vi "play-general-scan.vi"() -> ()   [LabVIEW 2017]
uses:
  fpga_VIs/fpga_subVIs_ssxy/fixed-point-ss/typeDefs/FXPControlParams-ss-xy.ctl
  controls/z-axis-params_v4_prescan.ctl
  controls/TF-params.ctl
  controls/scan_input_meta_data.ctl
  controls/scan-mode-CTL.ctl
  fpga_VIs/controls/supervisor-params.ctl
  fpga_VIs/controls/fpga-scan-status.ctl
  controls/boolean_info.ctl
  controls/auto_id_result.ctl
  subVIs/auto-sys-id/controls/SOS_frf_data.ctl
  fpga_interface_lib/fpga_interface_types/cs-scan-inputs-TYPE.ctl
  <vilib>/userdefined/High Color/nirio_resource_hc.ctl
  controls/rasterMetaData_asCS.ctl
  <vilib>/FPGAPlugInAG/cRIO-9082/niLvFpga_Open_cRIO-9082.vi
  <vilib>/rvi/interface/common/dynamic/niFpgaDynamicAddResources.vi
  <vilib>/FPGAPlugInAG/Dynamic/niLvFpga_Reset_Dynamic.vi
  <vilib>/Utility/error.llb/Error Cluster From Error Code.vi
  <vilib>/rvi/errors/niLvFpgaAdjustHostInterfaceError.vi
  <vilib>/FPGAPlugInAG/Dynamic/niLvFpga_Run_Dynamic.vi
  fpga_interface_lib/acquire_FXP_16-5_FIFO_2.vi
  <vilib>/RVI Host/nirviSupport.llb/nirviErrorClusterFromErrorCode.vi
  <vilib>/FPGAPlugInAG/Dynamic/niLvFpga_Close_Dynamic.vi
  <vilib>/rvi/interface/nirviOpenFPGA/nirviOpenFPGA.xnode
  FPGA Bitfiles/afmimagingcontro_FPGATargetSPARTA_cs-scanningv5ssx.lvbitx
  <vilib>/rvi/interface/nirviMethod/nirviMethod.xnode
  <vilib>/rvi/interface/nirviReadWriteControl/nirviReadWriteControl.xnode
  <vilib>/rvi/interface/nirviCloseFPGA/nirviCloseFPGA.xnode
  <vilib>/rvi/interface/Simulation/niFpgaSimulationCallBeginRW.vi
  NiFpgaLv.dll
  fpga_interface_lib/fpga_interface.lvlib
  <vilib>/addons/_JKI.lib/Serialization/JSON/JKI JSON Serialization.lvlib
  <vilib>/rvi/interface/nirviMethod/StockFPGA_InlinedMethodWaitForSingleIRQ.vi
  <vilib>/FPGAPlugInAG/Dynamic/niLvFpga_WaitOnIrq_Dynamic.vi
  <vilib>/FPGAPlugInAG/Dynamic/niLvFpga_AcknowledgeIrq_Dynamic.vi
  labview/utils_lib/utils.lvlib
panel:
  in  "enable-gdriftX":bool
  in  "enable-Dx":bool
  out "current-state":u8
  out "uy_k":fxp<+/-,32,5>
  in  "Ki-y":sgl=0.01
  in  "enable-Dy":bool=TRUE
  in  "Array 5":path[](array[path])
  out "size(s)":i32
  in  "log-channels":u16(ring)=6 items=["without-friction"=5, "with-friction"=6]
  in  "lpf-enable":bool=TRUE
  out "Array 3":T1(array[cluster])
  out "current-scan number":i32
  out "state0-count":u64
  out "output cluster":T2={"xy_settled_samples_threshold"=15, "xy_error_threshold"=0.01, "zup_err_threshold"=0.10000228881835938, "prescan_samples"=5000, "TOL"=0.3, "collect_all"=TRUE, "numEntities"=0} {"TOL" format="%#_13g"}
  out "error out":errorcluster
  in  "Alert-on-Finish":bool
  out "state times":dbl[](array[numeric])
  in  "Tab Control":T3(tab)
  in  "z_axis_params":T4={"z_u_max"=2.0, "setpoint_scan"=-0.3000030517578125, "Ki_scan"=0.07, "uz_safe"=0.2998046875, "Kiz_down"=0.045, "setpoint_up"=-0.8000030517578125, "do_Dz"=TRUE, "PID_while_xy_move"=FALSE, "TF_params"={"TF_order"=2, "Num"=[1.0, -1.9962076, 0.9990926, 0.0, 0.0, 0.0, 0.0, 0.0, 0.0], "Den"=[1.0, -1.9961313, 0.9990842, 0.0, 0.0, 0.0, 0.0, 0.0, 0.0]}, "KI_slope"=1.0, "enable_KI_sched"=FALSE, "KI_min"=0.0099945068359375, "KI_max"=0.1999969482421875} {"Kiz_down" format="%#_13g"; "Ki_scan" min=0 max=0.4 step=0.0025; "z_u_max" format="%#_13g"}
  in  "overwrite":bool
  in  "note-blob":string
  in  "state-machine-params":T2={"xy_settled_samples_threshold"=20, "xy_error_threshold"=0.01, "zup_err_threshold"=0.05100059509277344, "prescan_samples"=0, "TOL"=0.0259, "collect_all"=TRUE, "numEntities"=0} {"TOL" format="%#_13g"}
  in  "trigger-0":bool
  in  "STOP":bool
  out "CS Time":dbl
  in  "collect-0":bool
  in  "Continue":bool
  out "output-data-paths":path[](array[path])
  in  "file path (use dialog)":path=path "C:/Users/arnold/Documents/afm-cs/labview/first_res_fit_current.json"
  in  "xy-gain-mult":dbl=1.0 min=0.0 max=1.0 step=1.0 format="%#_13g"
  out "current-input-file":string
  in  "control_data_path":path=path "Z:/afm-cs/step-exps/LinControls-choose-zeta_5micron_xyff.json"
  in  "umax-xy":dbl=5.0 format="%#_13g"
  out "ControlParamsLin-ss":T6={"umax"=3.0, "Ns_obs/cntrl"=0, "du_max"=0.0, "Nbar"=0.0, "Nhyst"=0, "Nsat"=0, "Ndrift+1"=0, "Ki-y"=0.01, "Ns_xff+1"=0, "Ns_yff+1"=0, "Ns_Dx+1"=0, "Ns_Dy+1"=0, "Ki-x"=0.01}
  out "scan-status":T7
  out "error out 2":errorcluster
  out "scan_meta":T9
  out "Kiscan-effective":dbl
  out "Kidown-effective":dbl
  out "K":dbl
  out "last-state":u8[](array[numeric])
  out "Z-RESONANCE":T11
  out "input-file-check":bool[](array[boolean])
  out "output-meta-data-path":path
  # "C:\\Users\\arnold\\Documents\\afm-cs\\labview\\first_res_fit-4-19-2019-sicon.json"
  # "make this come from input csv!"
  # "For the y-axis only, shouldnt ever really\nneed to change"
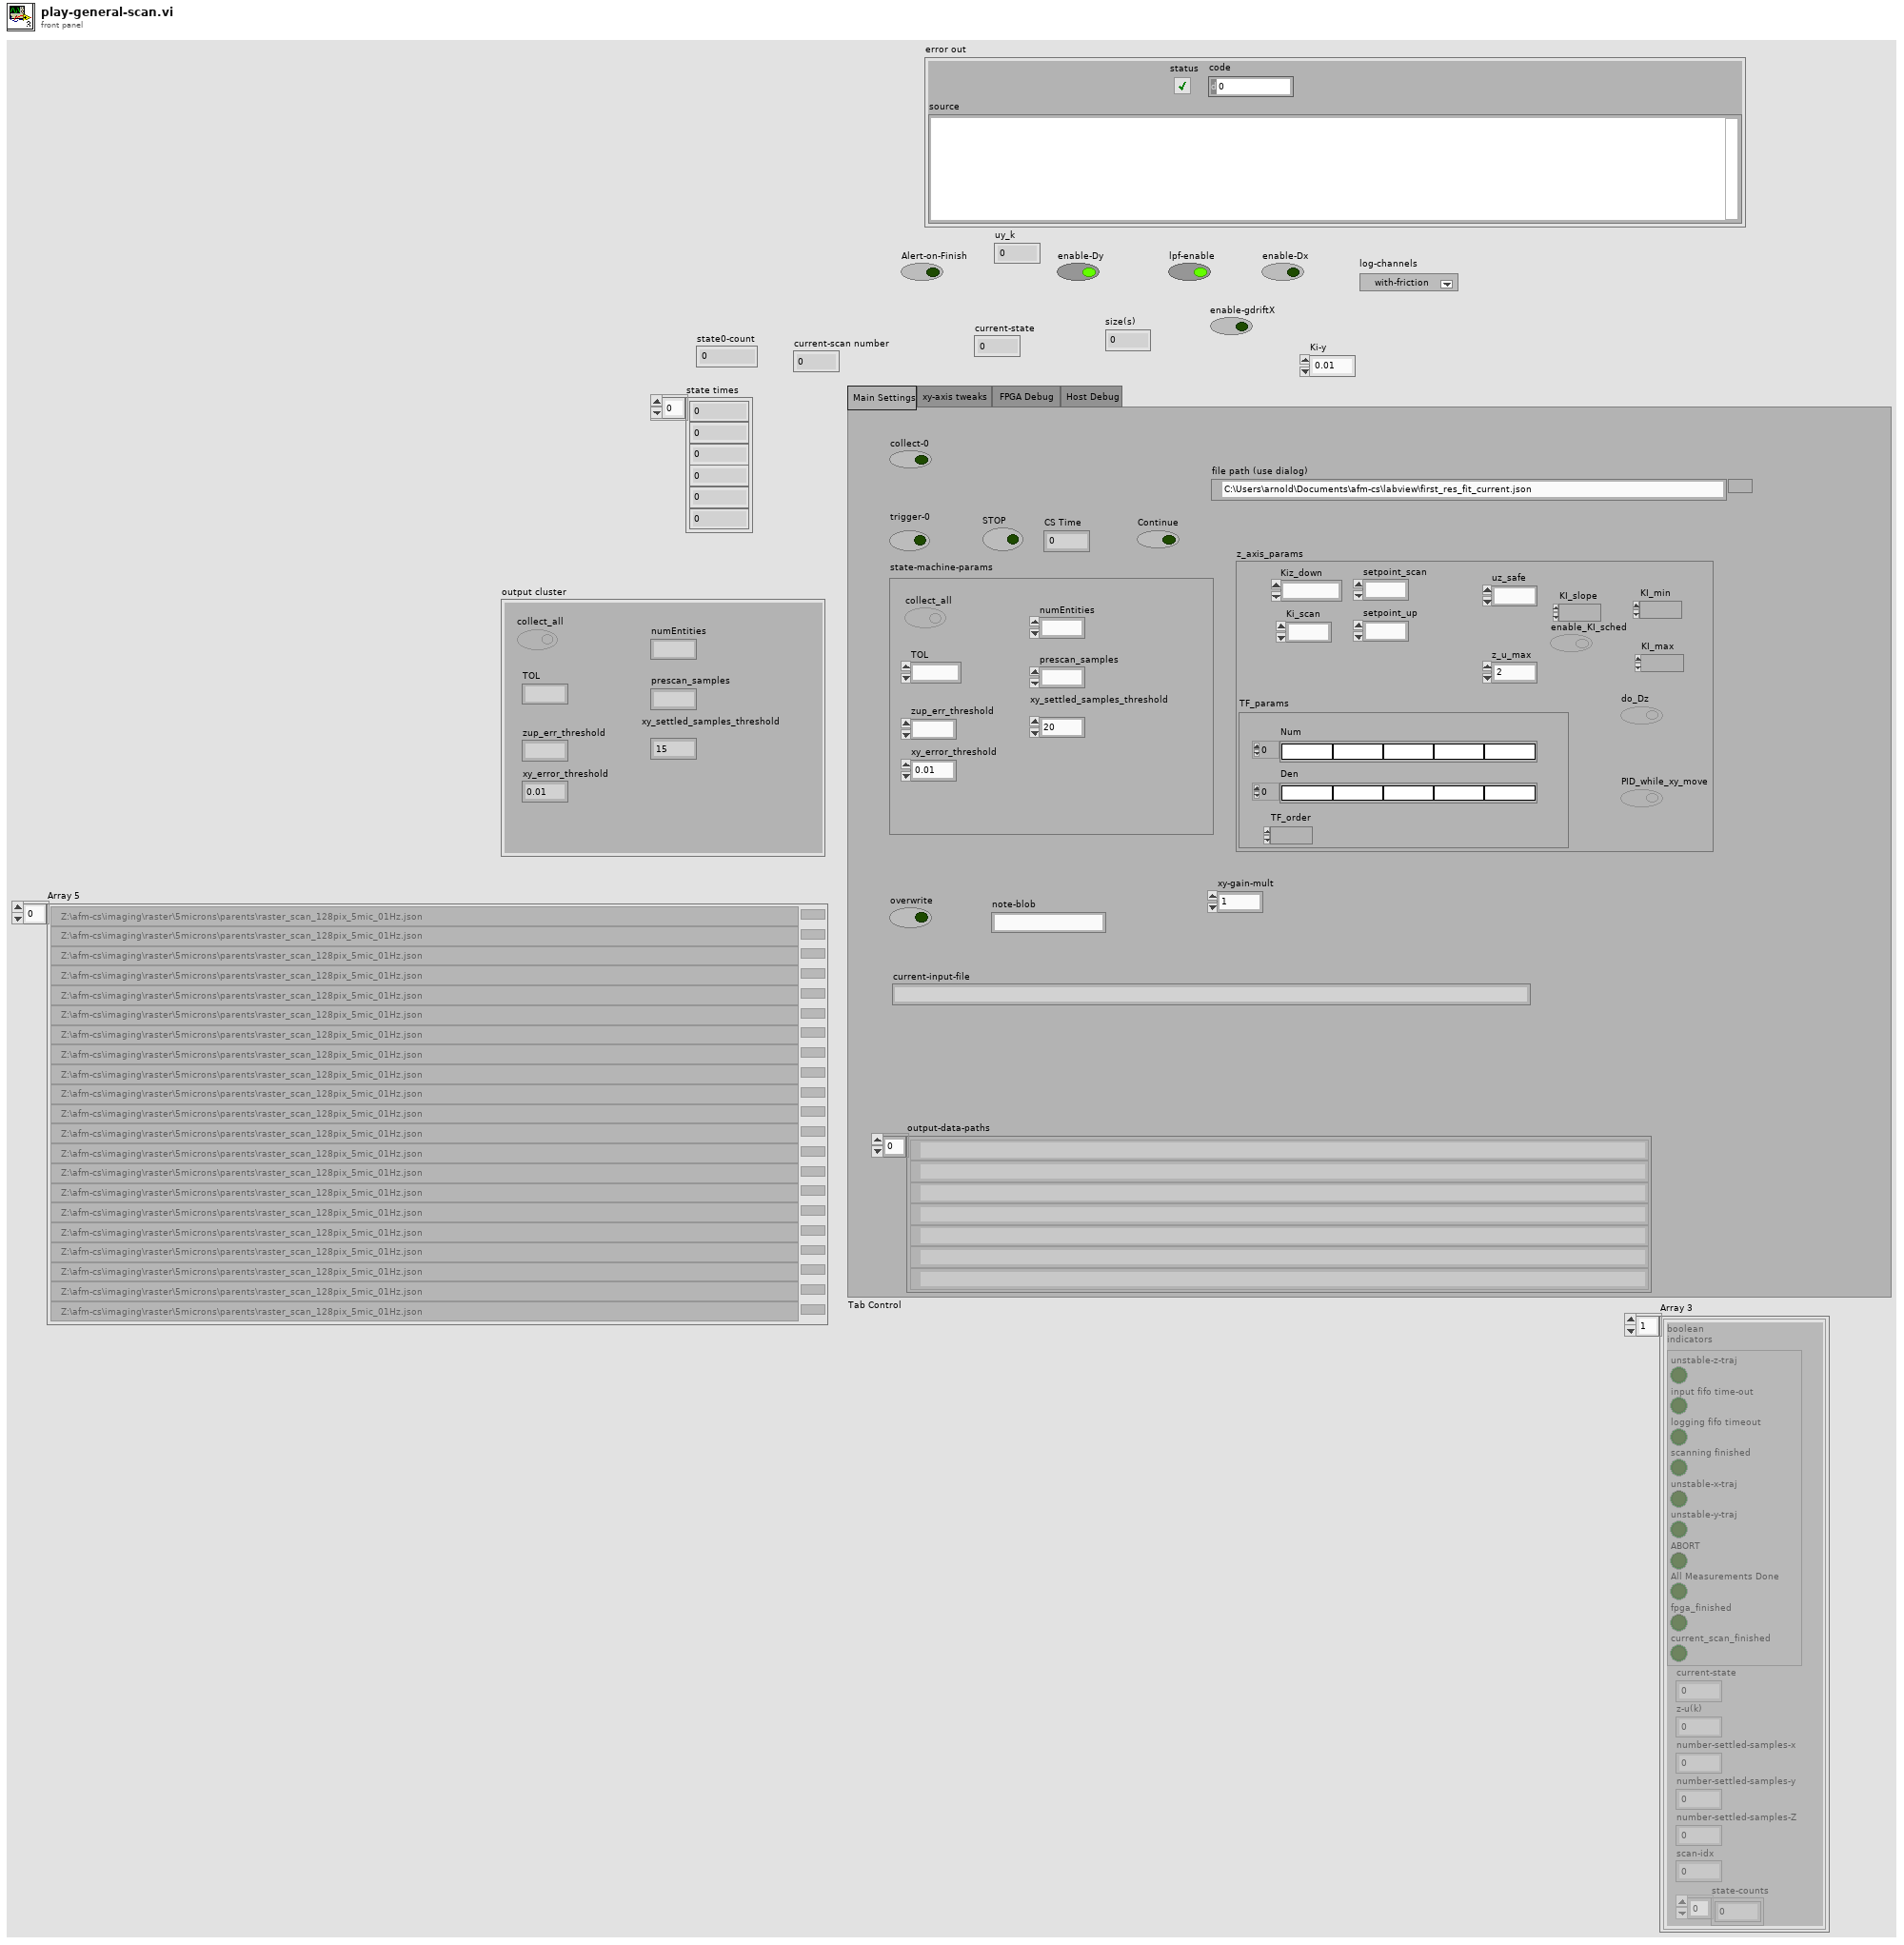
[diagram p1: front panel]
types:
  T1 = cluster{"boolean \nindicators":cluster{"unstable-z-traj":bool, "input fifo time-out":bool, "logging fifo timeout":bool, "scanning finished":bool, "unstable-x-traj":bool, "unstable-y-traj":bool, "ABORT":bool, "All Measurements Done":bool, "fpga_finished":bool, "current_scan_finished":bool}, "current-state":u8, "z-u(k)":sgl, "number-settled-samples-x":i16, "number-settled-samples-y":i16, "number-settled-samples-Z":i16, "scan-idx":i16, "state-counts":u64[]}[]
  T2 = typedef "supervisor-params.ctl" = cluster{"xy_settled_samples_threshold":i16, "xy_error_threshold":sgl, "zup_err_threshold":fxp<+,24,5>, "prescan_samples":i16, "TOL":sgl, "collect_all":bool, "numEntities":i16}
  T3 = enum32{"Main Settings", "xy-axis tweaks", "FPGA Debug ", "Host Debug"}
  T4 = typedef "z-axis-params_v4_prescan.ctl" = cluster{"z_u_max":sgl, "setpoint_scan":fxp<+/-,32,16>, "Ki_scan":sgl, "uz_safe":fxp<+/-,16,5>, "Kiz_down":sgl, "setpoint_up":fxp<+/-,32,16>, "do_Dz":bool, "PID_while_xy_move":bool, "TF_params":T5, "KI_slope":fxp<+/-,32,16>, "enable_KI_sched":bool, "KI_min":fxp<+/-,32,16>, "KI_max":fxp<+/-,32,16>}
  T5 = typedef "TF-params.ctl" = cluster{"TF_order":i16, "Num":sgl[], "Den":sgl[]}
  T6 = typedef "FXPControlParams-ss-xy.ctl" = cluster{"umax":fxp<+/-,18,5>, "Ns_obs/cntrl":u8, "du_max":fxp<+/-,18,5>, "Nbar":fxp<+/-,32,5>, "Nhyst":u8, "Nsat":u8, "Ndrift+1":u8, "Ki-y":sgl, "Ns_xff+1":u8, "Ns_yff+1":u8, "Ns_Dx+1":u8, "Ns_Dy+1":u8, "Ki-x":sgl}
  T7 = typedef "fpga-scan-status.ctl" = cluster{"boolean \nindicators":T8, "current-state":u8, "z-u(k)":sgl, "number-settled-samples-x":i16, "number-settled-samples-y":i16, "number-settled-samples-Z":i16, "scan-idx":i16, "state-counts":u64[]}
  T8 = typedef "boolean_info.ctl" = cluster{"unstable-z-traj":bool, "input fifo time-out":bool, "logging fifo timeout":bool, "scanning finished":bool, "unstable-x-traj":bool, "unstable-y-traj":bool, "ABORT":bool, "All Measurements Done":bool, "fpga_finished":bool, "current_scan_finished":bool}
  T9 = typedef "scan_input_meta_data.ctl" = cluster{"npix":i64, "raster_freq":dbl, "width":dbl, "points_per_line":i64, "points_per_period":i64, "total_num_points":i64, "scan_type":T10, "number_of_scans":i64, "actual_sub_samble_perc":dbl, "mu_length":dbl, "tip_velocity":dbl, "pix_idx":i32[], "overscan_samples":i16, "pre_scan_samples":i16}
  T10 = typedef "scan-mode-CTL.ctl" = enum16{"raster", "CS"}
  T11 = typedef "auto_id_result.ctl" = cluster{"Dinv_Num":dbl[], "SOS_frf_data":T12, "Dinv_den":dbl[], "K":dbl}
  T12 = typedef "SOS_frf_data.ctl" = cluster{"omegas":dbl[], "resp_real":dbl[], "resp_imag":dbl[], "theta0":dbl[]}
  T13 = enum16{"open", "replace", "create", "open or create", "replace or create", "replace or create with confirmation"}
  T14 = typedef "fpga_interface.lvlib/cs-scan-inputs-TYPE.ctl" = refnum<k20>
  T15 = typedef "nirio_resource_hc.ctl" = tag
  T16 = typedef "rasterMetaData_asCS.ctl" = cluster{"Ki_xy":dbl, "number_of_lines":i32, "Ki_derate":sgl, "ze_sched_thresh":sgl, "scan_meta":T9, "z_axis_params":T4, "state_counts":dbl[], "state_machine_params":T2, "input_data_path":path, "output_data_path":path, "xy_control_path":path}
  T17 = cluster{"boolean \nindicators":cluster{"unstable-z-traj":bool, "input fifo time-out":bool, "logging fifo timeout":bool, "scanning finished":bool, "unstable-x-traj":bool, "unstable-y-traj":bool, "ABORT":bool, "All Measurements Done":bool, "fpga_finished":bool, "current_scan_finished":bool}, "current-state":u8, "z-u(k)":sgl, "number-settled-samples-x":i16, "number-settled-samples-y":i16, "number-settled-samples-Z":i16, "scan-idx":i16, "state-counts":u64[]}
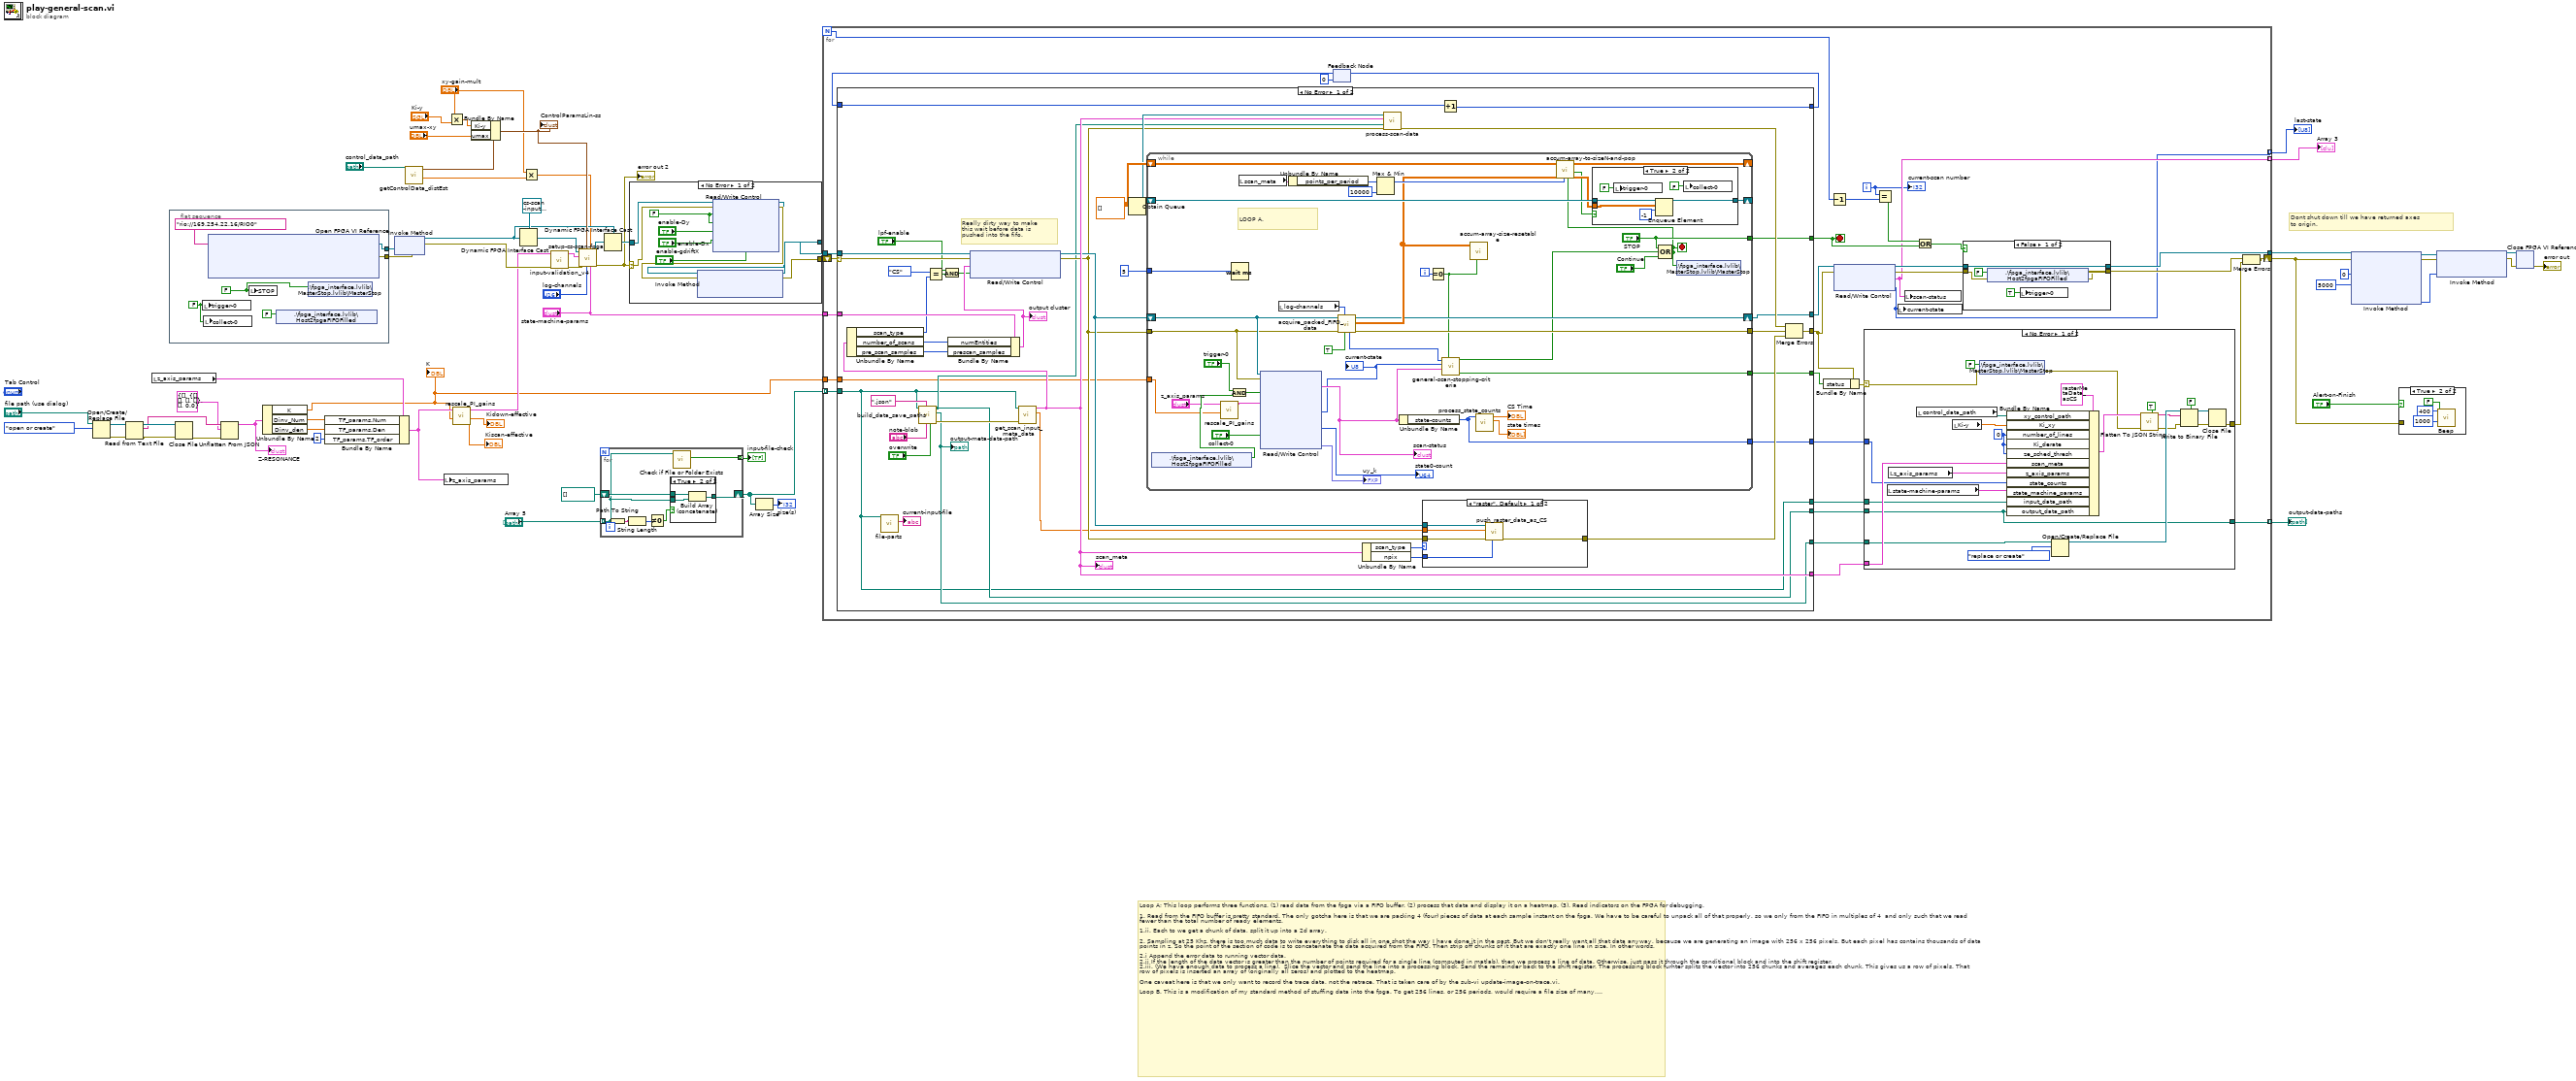
[diagram p0: block diagram]
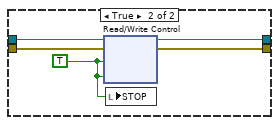
[diagram p4: hidden frame]
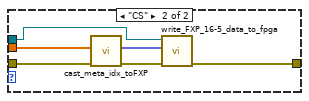
[diagram p6: hidden frame]
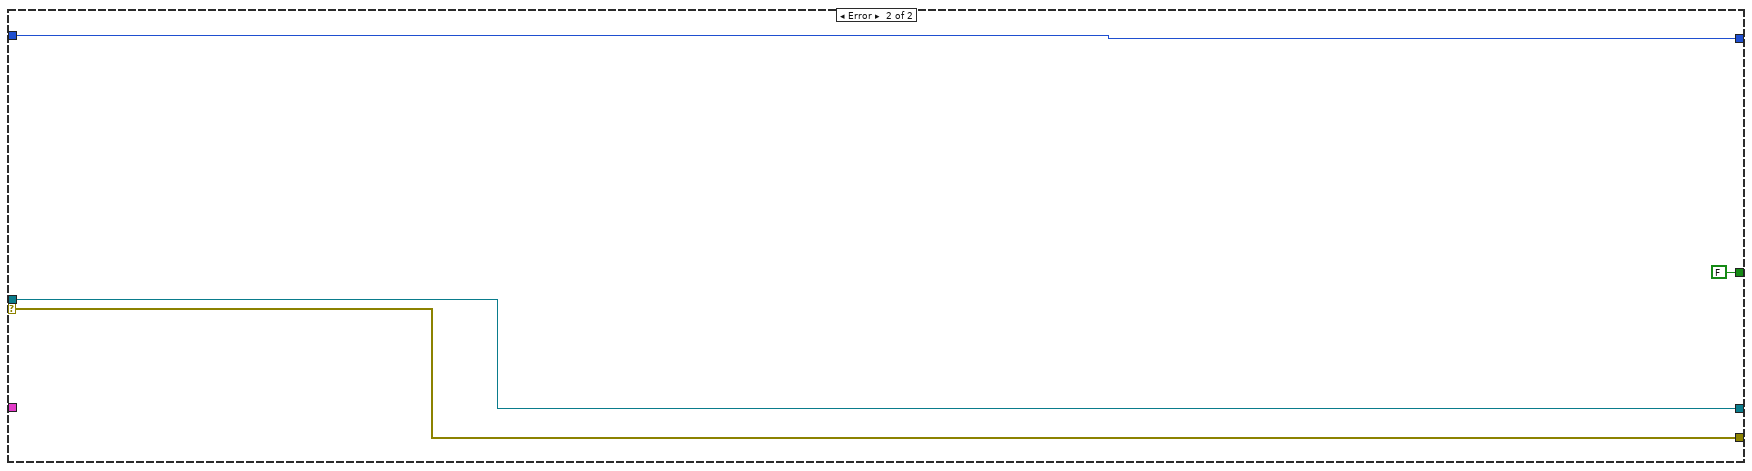
[diagram p8: hidden frame]
diagram:
  # "Dont shut down till we have returned axes\nto origin."
  # "Loop A; This loop performs three functions. (1) read data from the fpga via a FIFO buffer. (2) process that data and display it on a heatmap. (3). Read indicators on the FPGA for debugging.\n\n1. Read from the FIFO buffer is pretty standard. The only gotcha here is that we are packing 4 (four) pieces of data at each sample instant on the fpga. We have to be careful to unpack all of that properly, so we only from the FIFO in multiples of 4  and only such that we read fewer than the total number of ready elements. \n\n1.ii. Each to we get a chunk of data, split it up into a 2d array. \n\n2. Sampling at 25 Khz, there is too much data to write everything to disk all in one shot the way I have done it in the past. But we don't really want all that data anyway, because we are generating an image with 256 x 256 pixels. But each pixel has contains thousands of data points in z. So the point of the section of code is to concatenate the data acquired from the FIFO. Then strip off chunks of it that are exactly one line in size. In other words,\n\n2.i Append the error data to running vector data.\n2.ii If the length of the data vector is greater than the number of points required for a single line (computed in matlab), then we process a line of data. Otherwise, just pass it through the conditional block and into the shift register. \n2.iii. (We have enough data to process a line).  Slice the vector and send the line into a processing block. Send the remainder back to the shift register. The processing block furhter splits the vector into 256 chunks and averages each chunk. This gives us a row of pixels. That row of pixels is inserted an array of (originally all zeros) and plotted to the heatmap.\n\nOne caveat here is that we only want to record the trace data, not the retrace. That is taken care of by the sub-vi update-image-on-trace.vi.\n\nLoop B. This is a modification of my standard method of stuffing data into the fpga. To get 256 lines, or 256 periods, would require a file size of many, many gigibtyes. SO the point here is to only use a single period of the triangle wave and corresponding ramp signal. Everytime we exauhst that data, re-cycle the same data and keep pumping it back in. The one tricky part here is that we have to be careful to shift the original ramp data up by the appropriate amount. We also have to take special care because of how the data is packed from matlab. [x(1), y(1), x(2), y(2)...].\n\nThe first iteration of the loop, we don't push any data in. All we do is get the number of empty elements.\n\nB.1 Each iteration, strip off ' empty elements ' elements from the array and send them to FIFO. \nB.2.i Is the remaining array empty?\nB.2.ii Grab the very last element. We need this"
  n1 = Open/Create/Replace File(file path (use dialog)="file path (use dialog)", operation (0:open)=T13."open or create") -> (refnum out=w34:refnum<file>, error out=w35:errorcluster)  [unwired: 4 in, 1 out]
  n2 = Read from Text File(file (use dialog)=w34, error in=w35) -> (refnum out=w33:refnum<file>, text=w31:string, error out=w32:errorcluster)  [unwired: 2 in, 1 out]
  n3 = local read "z_axis_params"() -> (w23:T4)
  n4 = flat-sequence {
    tunnel: [w68] -> w62
    tunnel: [w67] -> w61
    frame #0 {
      w63 = FALSE ("trigger-0")
      w65 = FALSE
      n5 = local write "trigger-0"(w63) -> ()
      n6 = local write "collect-0"(w63) -> ()
      n7 = xnode "Open FPGA VI Reference"("resource name"=T15 "rio://169.254.22.16/RIO0") -> ("FPGA VI Reference Out"=w68:refnum<k20>, "error out"=w67:errorcluster)  [unwired: 1 in]
      n8 = local write "STOP"(w65) -> ()
      n9 = shared-variable ".\\fpga_interface.lvlib\\Host2fpgaFIFOFilled"(FALSE ("Host2fpgaFIFOFilled")) -> ()  [unwired: 1 in, 1 out]
      n10 = shared-variable ".\\fpga_interface.lvlib\\MasterStop.lvlib\\MasterStop"(w65) -> ()  [unwired: 1 in, 1 out]
    }
  }
  n11 = Close File(refnum=w33, error in=w32) -> (error out=w30:errorcluster)  [unwired: 1 out]
  n12 = Unflatten From JSON(JSON string=w31, type and defaults=T11 {"Dinv_Num"=[], "SOS_frf_data"={"omegas"=[], "resp_real"=[], "resp_imag"=[], "theta0"=[]}, "Dinv_den"=[], "K"=0.0} ("auto_id_result 2"), error in (no error)=w30) -> (value=w27:T11)  [unwired: 4 in, 1 out]
  "Z-RESONANCE" <- w27
  n13 = Unbundle By Name(w27) -> ("K"=w12:dbl, "Dinv_Num"=w22:dbl[], "Dinv_den"=w26:dbl[])
  "K" <- w12
  n14 = Bundle By Name(cluster=w23, "TF_params.Num"=w22, "TF_params.Den"=w26, "TF_params.TF_order"=i16 2) -> (w15:T4)
  n15 = xnode "Invoke Method"("FPGA VI Reference In"=w62, "error in"=w61) -> ("FPGA VI Reference Out"=w21:refnum<k20>, "error out"=w41:errorcluster)
  n16 = call "getControlData_distEst.vi"("system data path"="control_data_path") -> ("AllMatrix"=w11:dbl[], "ControlParams"=w59:T6)  [unwired: 7 in, 2 out]
  n17 = local write "z_axis_params"(w15) -> ()
  n18 = Multiply(x="xy-gain-mult", y="Ki-y") -> (x*y=w9:dbl)
  n19 = call "rescale_PI_gains.vi"("Dinv-k"=w12, "z-axis-params-in"=w15) -> ("Kiscan-effective"=→"Kiscan-effective":dbl, "Kidown-effective"=→"Kidown-effective":dbl, "z-axis-params-out"=w16:T4)  [unwired: 7 in]
  n20 = Bundle By Name(cluster=w59, "Ki-y"=w9, "umax"="umax-xy") -> (w42:T6)
  "ControlParamsLin-ss" <- w42
  n21 = Dynamic FPGA Interface Cast(Session In=T14 refnum ("FPGA Interface in"), Type=w21) -> (Session Out=w44:T14)
  n22 = Multiply(x="xy-gain-mult", y=w11) -> (x*y=w10:dbl[])
  n23 = call "input-validation_v4.vi"("error constant"=w41, "z_axis_params"=w16) -> ("error out"=w25:errorcluster, "z_axis_params-out"=w5:T4)  [unwired: 8 in]
  n24 = call "setup-cs-scan-fpga.vi"("state-machine-params"="state-machine-params", "Control-matrices"=w10, "log-channels"="log-channels", "ControlParamsLin-ss"=w42, "error in"=w25, "z_axis_params"=w5, "FPGA Interface in"=w44) -> ("error out"=w24:errorcluster, "FPGA Interface out"=w39:T14)  [unwired: 3 in]
  "error out 2" <- w24
  n25 = for {
    tunnel: "Array 5" -> [w70] mode=indexing
    shift-right: [w73] -> w3
    shift-left: path[] [] -> [w74]
    tunnel: [w69] -> w4 mode=indexing
    n26 = Path To String(path=w70) -> (string=w75:string)
    n27 = String Length(string=w75) -> (length=w71:i32)
    n28 = Not Equal To 0?(x=w71) -> (x != 0?=w72:bool)
    n29 = case shown="True" w72 {
      tunnel: w74 -> [w76 w78]
      tunnel: [w76 w79] -> w73
      tunnel: w70 -> [_ w77]
      frame False {
      }
      frame True {
        n30 = Build Array (concatenate)(w78, w77) -> (w79:path[])
      }
    }
    n31 = call <vilib>:"Check if File or Folder Exists.vi"("path"=w70) -> ("file or folder exists?"=w69:bool)  [unwired: 8 in, 2 out]
  }
  "input-file-check" <- w4
  n32 = Dynamic FPGA Interface Cast(Session In=w21, Type=w39) -> (Session Out=w40:refnum<k20>)
  n33 = case shown="No Error" w24 {
    selector: w24 -> [w85 w90]
    tunnel: w40 -> [w86 w91]
    tunnel: [w89 w90] -> w57
    tunnel: [w88 w91] -> w56
    frame No Error {
      w83 = FALSE ("trigger-0")
      n34 = xnode "Read/Write Control"("FPGA VI Reference In"=w86, "error in"=w85, "trigger-0"=w83, "lpf-enable"=w83, "enable-Dy"="enable-Dy", "enable-Dx"="enable-Dx", "enable-gdriftX"="enable-gdriftX") -> ("FPGA VI Reference Out"=w84:refnum<k20>, "error out"=w87:errorcluster)
      n35 = xnode "Invoke Method"("FPGA VI Reference In"=w84, "error in"=w87) -> ("FPGA VI Reference Out"=w88:refnum<k20>, "error out"=w89:errorcluster)  [unwired: 1 in]
    }
    frame Error {
    }
  }
  n36 = Array Size(array=w3) -> (size(s)=→"size(s)":i32)
  n37 = for {
    N -> [w104]
    shift-right: [w112] -> w47
    shift-left: w57 -> [w121]
    tunnel: w56 -> [w120]
    tunnel: [w113] -> w45
    tunnel: "state-machine-params" -> [w108]
    tunnel: w3 -> [w105] mode=indexing
    tunnel: [w100] -> w19 mode=indexing
    tunnel: [w99] -> w20 mode=indexing
    tunnel: [w97] -> w18 mode=indexing
    tunnel: w12 -> [w93]
    i -> [w92]
    stop <- w117 stop-if-true
    n38 = feedback #1(i16 0) -> (w102:i16)
    n39 = case shown="No Error" w121 {
      selector: w121 -> [w180 w257]
      tunnel: [w195 w257] -> w96
      tunnel: [w186 w258] -> w119
      tunnel: w120 -> [w181 w258]
      tunnel: [w176 _] -> w123
      tunnel: [w188 _] -> w122
      tunnel: [w187 FALSE ("STOP")] -> w117
      tunnel: w108 -> [w170 _]
      tunnel: w105 -> [w160 _]
      tunnel: [w160 _] -> w107
      tunnel: [w175 _] -> w106
      tunnel: [w172 w256] -> w103
      tunnel: w102 -> [w171 w256]
      tunnel: [w169 _] -> w98
      tunnel: [w168 _] -> w94
      tunnel: w93 -> [w167 _]
      frame No Error {
        w193 = dbl[][] []
        # "Really dirty way to make\nthis wait before data is\npushed into the fifo."
        n40 = call "file-parts.vi"("full-path-file"=w160) -> ("file-name"=→"current-input-file":string)  [unwired: 8 in, 2 out]
        n41 = call "build_data_save_paths.vi"("overwrite"="overwrite", "note-blob"="note-blob", "meta-file-ext"=".json" ("replace string (\"\")"), "input-file"=w160) -> ("error IO"=w185:errorcluster, "output-meta-data-path"=w175:path, "output-data-path"=w169:path)  [unwired: 4 in, 1 out]
        "output-meta-data-path" <- w175
        n42 = call "get_scan_input_meta_data.vi"("error in"=w185, "Path"=w160) -> ("fpga_input"=w166:dbl[], "meta_data"=w176:T9)  [unwired: 7 in, 1 out]
        "scan_meta" <- w176
        n43 = Unbundle By Name(w176) -> ("scan_type"=w164:T10, "number_of_scans"=w178:i64, "pre_scan_samples"=w179:i16)
        n44 = Equal?(x=scan-mode-CTL."CS" ("scan_type"), y=w164) -> (x = y?=w163:bool)
        n45 = And(x="lpf-enable", y=w163) -> (x .and. y?=w162:bool)
        n46 = Bundle By Name(cluster=w170, "numEntities"=w178, "prescan_samples"=w179) -> (w177:T2)
        "output cluster" <- w177
        n47 = xnode "Read/Write Control"("FPGA VI Reference In"=w181, "error in"=w180, "state-machine-params"=w177, "lpf-enable"=w162) -> ("FPGA VI Reference Out"=w174:refnum<k20>, "error out"=w173:errorcluster)
        n48 = Obtain Queue(element data type=w193) -> (queue out=w191:refnum<queue>)  [unwired: 4 in, 2 out]
        n49 = while {
          tunnel: 5 -> [w248]
          tunnel: [w245] -> w196
          shift-right: [w247] -> _
          shift-left: w191 -> [w246]
          tunnel: w173 -> [w227]
          tunnel: [w233] -> w188
          shift-right: [w241] -> _
          shift-left: w193 -> [w240]
          tunnel: ["STOP"] -> w187
          shift-right: [w230] -> w186
          shift-left: w174 -> [w228]
          tunnel: [w215] -> w168
          tunnel: w167 -> [w211]
          i -> [w231]
          stop <- w214 stop-if-true
          # "LOOP A."
          n50 = shared-variable ".\\fpga_interface.lvlib\\Host2fpgaFIFOFilled"() -> (w223:bool)  [unwired: 1 in, 1 out]
          n51 = call "rescale_PI_gains.vi"("Dinv-k"=w211, "z-axis-params-in"="z_axis_params") -> ("z-axis-params-out"=w213:T4)  [unwired: 7 in, 2 out]
          n52 = And(x="trigger-0", y=w223) -> (x .and. y?=w226:bool)
          n53 = Wait (ms)(milliseconds to wait=w248) -> ()  [unwired: 1 out]
          n54 = local read "scan_meta"() -> (w237:T9)
          n55 = xnode "Read/Write Control"("FPGA VI Reference In"=w228, "error in"=w227, "trigger-0"=w226, "z_axis_params"=w213, "collect-0"="collect-0") -> ("scan-status"=w221:T17, "current-state"=w220:u8, "state0-count"=→"state0-count":u64, "uy_k"=→"uy_k":fxp<+/-,32,5>)  [unwired: 3 out]
          "scan-status" <- w221
          "current-state" <- w220
          n56 = local read "log-channels"() -> (w210:u16)
          n57 = Unbundle By Name(w237) -> ("points_per_period"=w236:i64)
          n58 = call-poly "acquire_packed_FIFO_data.vi"("Run once?"=TRUE, "numChannels"=w210, "error in"=w227, "FPGA Interface(in)"=w228) -> ("error out"=w245:errorcluster, "2D Data Out"=w232:dbl[][], "FPGA VI Reference Out"=w230:refnum<k20>, "Elements Remaining"=w219:u32)  [unwired: 3 in, 1 out]
          n59 = Max & Min(x=w236, y=i64 10000) -> (max(x,y)=w234:i64)  [unwired: 1 out]
          n60 = Unbundle By Name(w221) -> ("state-counts"=w233:u64[])
          n61 = Equal To 0?(x=w231) -> (x = 0?=w218:bool)
          n62 = call "general-scan-stopping-criteria.vi"("reset"=w218, "scan-status"=w221, "current-state"=w220, "FIFO-elementas-left"=w219) -> ("FIFO timeout"=w215:bool, "Finish"=w217:bool)  [unwired: 6 in]
          n63 = call "accum-array-size-resetable.vi"("reset"=w218, "array"=w232) -> ()  [unwired: 9 in, 1 out]
          n64 = call "process_state_counts.vi"("state-counts"=w233) -> ("State_times"=→"state times":dbl[], "Cs_time"=→"CS Time":dbl)  [unwired: 9 in]
          n65 = Compound Arithmetic op=OR("STOP", w217, "Continue") -> (w214:bool)
          n66 = call "accum-array-to-sizeN-and-pop.vi"("flush"=w214, "Nsize"=w234, "new-data-in"=w232, "old-data-in"=w240) -> ("popped-data"=w239:dbl[][], "new-data-ready"=w238:bool, "old-data-out"=w241:dbl[][])  [unwired: 5 in]
          n67 = case shown="True" w238 {
            tunnel: w246 -> [w249 w255]
            tunnel: w239 -> [_ w253]
            tunnel: [w249 w252] -> w247
            frame False {
            }
            frame True {
              n68 = local write "trigger-0"(FALSE ("trigger-0")) -> ()
              n69 = Enqueue Element(queue=w255, element=w253, timeout in ms (-1)=-1) -> (queue out=w252:refnum<queue>)  [unwired: 1 in, 2 out]
              n70 = local write "collect-0"(FALSE ("collect-0")) -> ()
            }
          }
          n71 = shared-variable ".\\fpga_interface.lvlib\\MasterStop.lvlib\\MasterStop"(w214) -> ()  [unwired: 1 in, 1 out]
        }
        n72 = Unbundle By Name(w176) -> ("scan_type"=w189:T10, "npix"=w192:i64)
        n73 = call "process-scan-data.vi"("error in"=w173, "output-data-path"=w169, "scan_meta"=w176, "queue in"=w191) -> ("error out"=w190:errorcluster)  [unwired: 7 in]
        n74 = case shown="\"raster\", Default" w189 {
          tunnel: [w202 w208] -> w194
          tunnel: w174 -> [w201 w203]
          tunnel: w192 -> [w200 _]
          tunnel: w173 -> [w199 w207]
          tunnel: w166 -> [w198 w204]
          frame "raster", Default {
            n75 = call "push_raster_data_as_CS.vi"("number-of-pixels"=w200, "error in"=w199, "fpga_input_vec"=w198, "FPGA Interface"=w201) -> ("error out"=w202:errorcluster)  [unwired: 6 in, 1 out]
          }
          frame "CS" {
            n76 = call "cast_meta_idx_toFXP.vi"("error in"=w207, "cs-traj-data-in"=w204) -> ("error out"=w206:errorcluster, "cs-traj-data-out"=w205:fxp<+/-,16,5>[])  [unwired: 8 in]
            n77 = call "write_FXP_16-5_data_to_fpga.vi"("error in"=w206, "all rows"=w205, "FPGA Interface"=w203) -> ("error out"=w208:errorcluster)  [unwired: 7 in, 1 out]
          }
        }
        n78 = Increment(x=w171) -> (x+1=w172:i16)
        n79 = Merge Errors(w190, w196, w194) -> (w195:errorcluster)
      }
      frame Error {
      }
    }
    n80 = feedback-in #1(w103) -> ()
    n81 = Bundle By Name(cluster=w96, "status"=w94) -> (w95:errorcluster)
    n82 = Decrement(x=w104) -> (x-1=w109:i32)
    n83 = xnode "Read/Write Control"("FPGA VI Reference In"=w119, "error in"=w96) -> ("FPGA VI Reference Out"=w115:refnum<k20>, "error out"=w114:errorcluster, "scan-status"=w100:T17, "current-state"=w99:u8)
    n84 = case shown="No Error" w95 {
      selector: w95 -> [w139 w158]
      tunnel: w123 -> [w150 _]
      tunnel: w122 -> [w142 _]
      tunnel: [w141 w158] -> w111
      tunnel: w107 -> [w136 _]
      tunnel: w106 -> [w137 _]
      tunnel: w98 -> [w135 _]
      tunnel: [w135 _] -> w97
      frame No Error {
        w143 = 0 ("number_of_lines")
        n85 = local read "state-machine-params"() -> (w145:T2)
        n86 = local read "z_axis_params"() -> (w146:T4)
        n87 = local read "control_data_path"() -> (w134:path)
        n88 = local read "Ki-y"() -> (w144:sgl)
        n89 = shared-variable ".\\fpga_interface.lvlib\\MasterStop.lvlib\\MasterStop"(FALSE ("MasterStop"), error in=w139) -> (error out=w138:errorcluster)
        n90 = Bundle By Name(cluster=T16 {"Ki_xy"=7.0, "number_of_lines"=0, "Ki_derate"=0.01, "ze_sched_thresh"=0.0, "scan_meta"={"npix"=0, "raster_freq"=0.0, "width"=0.0, "points_per_line"=0, "points_per_period"=0, "total_num_points"=0, "scan_type"=enum."raster", "number_of_scans"=0, "actual_sub_samble_perc"=0.0, "mu_length"=0.0, "tip_velocity"=0.0, "pix_idx"=[], "overscan_samples"=0, "pre_scan_samples"=0}, "z_axis_params"={"z_u_max"=5.0, "setpoint_scan"=-0.3000030517578125, "Ki_scan"=0.02, "uz_safe"=0.0, "Kiz_down"=0.02, "setpoint_up"=-0.899993896484375, "do_Dz"=FALSE, "PID_while_xy_move"=FALSE, "TF_params"={"TF_order"=0, "Num"=[0.0, 0.0, 0.0, 0.0, 0.0, 0.0, 0.0, 0.0, 0.0], "Den"=[0.0, 0.0, 0.0, 0.0, 0.0, 0.0, 0.0, 0.0, 0.0]}, "KI_slope"=0.0, "enable_KI_sched"=FALSE, "KI_min"=0.0, "KI_max"=0.0}, "state_counts"=[], "state_machine_params"={"xy_settled_samples_threshold"=0, "xy_error_threshold"=0.01, "zup_err_threshold"=0.0, "prescan_samples"=-12144, "TOL"=256.0, "collect_all"=TRUE, "numEntities"=256}, "input_data_path"=path "", "output_data_path"=path "", "xy_control_path"=path ""} ("raster_asCS__meta_out"), "xy_control_path"=w134, "Ki_xy"=w144, "number_of_lines"=w143, "Ki_derate"=w143, "ze_sched_thresh"=w143, "scan_meta"=w150, "z_axis_params"=w146, "state_counts"=w142, "state_machine_params"=w145, "input_data_path"=w136, "output_data_path"=w135) -> (w147:T16)
        n91 = Open/Create/Replace File(file path (use dialog)=w137, operation (0:open)=T13."replace or create") -> (refnum out=w154:refnum<file>)  [unwired: 4 in, 2 out]
        n92 = call <vilib>:"Flatten To JSON String.vi"("Numeric Extensions (F)"=TRUE, "error in (no error)"=w138, "Variant"=w147) -> ("error out"=w151:errorcluster, "JSON String"=w152:string)  [unwired: 7 in]
        n93 = Write to Binary File(file (use dialog)=w154, data=w152, error in=w151, 5:FALSE ("prepend array or string size? (T)")) -> (refnum out=w155:refnum<file>, error out=w156:errorcluster)  [unwired: 2 in, 1 out]
        n94 = Close File(refnum=w155, error in=w156) -> (error out=w141:errorcluster)  [unwired: 1 out]
      }
      frame Error {
      }
    }
    n95 = Equal?(x=w92, y=w109) -> (x = y?=w118:bool)
    n96 = local write "current-state"(w99) -> ()
    n97 = local write "scan-status"(w100) -> ()
    n98 = Or(x=w118, y=w117) -> (x .or. y?=w116:bool)
    n99 = case shown="False" w116 {
      tunnel: w115 -> [w128 w133]
      tunnel: w114 -> [w126 w132]
      tunnel: [w128 w131] -> w113
      tunnel: [w125 w130] -> w110
      frame False {
        n100 = shared-variable ".\\fpga_interface.lvlib\\Host2fpgaFIFOFilled"(FALSE ("Host2fpgaFIFOFilled"), error in=w126) -> (error out=w125:errorcluster)
        n101 = local write "trigger-0"(TRUE ("trigger-0")) -> ()
      }
      frame True {
        w129 = TRUE ("ABORT")
        n102 = xnode "Read/Write Control"("FPGA VI Reference In"=w133, "error in"=w132, "ABORT"=w129, "stop"=w129) -> ("FPGA VI Reference Out"=w131:refnum<k20>, "error out"=w130:errorcluster)
        n103 = local write "STOP"(w129) -> ()
      }
    }
    n104 = Merge Errors(w110, w111) -> (w112:errorcluster)
    "current-scan number" <- w92
  }
  "last-state" <- w20
  "Array 3" <- w19
  "output-data-paths" <- w18
  n105 = xnode "Invoke Method"("FPGA VI Reference In"=w45, "error in"=w47, "IRQ Number(s)"=0, "Timeout (ms)"=5000) -> ("FPGA VI Reference Out"=w54:refnum<k20>, "error out"=w53:errorcluster, "IRQ(s) Asserted"=w55:i32)  [unwired: 1 out]
  n106 = case shown="True" "Alert-on-Finish" {
    tunnel: w47 -> [_ _]
    frame False {
    }
    frame True {
      n107 = call <vilib>:"Beep.vi"("use system alert? (T)"=FALSE, "duration (msec)"=u32 1000, "frequency (Hz)"=u32 400) -> ()  [unwired: 9 in]
    }
  }
  n108 = xnode "Invoke Method"("FPGA VI Reference In"=w54, "error in"=w53, "IRQ Number(s)"=w55) -> ("FPGA VI Reference Out"=w50:refnum<k20>, "error out"=w49:errorcluster)
  n109 = xnode "Close FPGA VI Reference"("FPGA VI Reference In"=w50, "error in"=w49) -> ("error out"=→"error out":errorcluster)
